vi "Set Frequency.vi"(8 "error in (no error)":errorcluster, 9 "Synchronous":bool, 10 "Frequency":dbl format="%#_6pHz", 11 "Red Pitaya Lock-in Driver in":refnum<class "Red Pitaya Lock-in Driver.lvclass">) -> (0 "error out":errorcluster, 2 "Actual frequency":dbl format="%#_6pHz", 3 "Red Pitaya Lock-in Driver out":refnum<class "Red Pitaya Lock-in Driver.lvclass">)   [LabVIEW 2016, in "Red Pitaya Lock-in Driver.lvclass"]
uses:
  Red Pitaya Lock-in Driver.lvclass
  Red Pitaya Lock-in Driver.lvclass/Red Pitaya Lock-in Driver.ctl
  Read RP Instrument.vi
  Write RP Instrument.vi
  RP Instrument/RP Instrument.lvclass
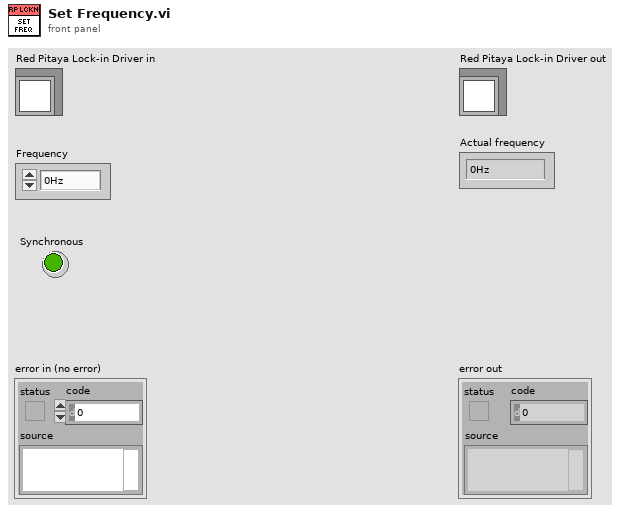
[diagram p1: front panel]
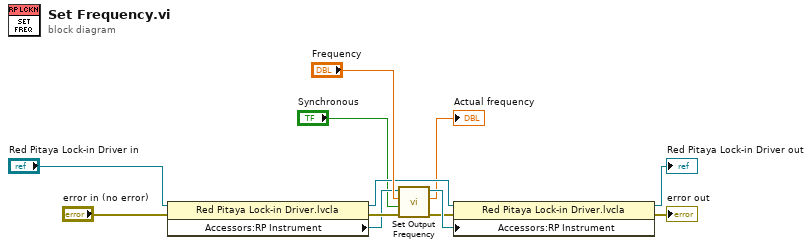
[diagram p0: block diagram]
diagram:
  n1 = property class="Red Pitaya Lock-in Driver.lvcla"(reference="Red Pitaya Lock-in Driver in", error in="error in (no error)") -> (reference out=w9:refnum<class "Red Pitaya Lock-in Driver.lvclass">, error out=w4:errorcluster, "Accessors:RP Instrument"=w2:refnum<class "RP Instrument.lvclass">)
  n2 = call-dynamic "Set Output Frequency.vi"("error in (no error)"=w4, "Synchronous"="Synchronous", "Frequency"="Frequency", "RP Instrument in"=w2) -> ("error out"=w5:errorcluster, "Actual frequency"=→"Actual frequency":dbl, "RP Instrument out"=w8:refnum<class "RP Instrument.lvclass">)  [unwired: 5 in]
  n3 = property class="Red Pitaya Lock-in Driver.lvcla"(reference=w9, error in=w5, "Accessors:RP Instrument"=w8) -> (reference out=→"Red Pitaya Lock-in Driver out":refnum<class "Red Pitaya Lock-in Driver.lvclass">, error out=→"error out":errorcluster)
